vi "G#Interface_ExecuteVI.vi"(0 "reference in":refnum<class "G#Interface.lvclass">, 2 "VI Refnum":refnum<vi>, 5 "error in (no error)":errorcluster) -> (14 "reference out":refnum<class "G#Interface.lvclass">, 19 "error out":errorcluster)   [LabVIEW 2020, in "G#Interface.lvclass"]
uses:
  G#Interface.lvclass
  C:/ProjectGSharpDevelopment_2020-3/gsharp/VIPM/Files/vi.lib/addons/_AddQ/G#Object/G#Object.lvclass
  G#Interface.lvclass/G#Interface.ctl
  G#Object/G#Object.lvclass
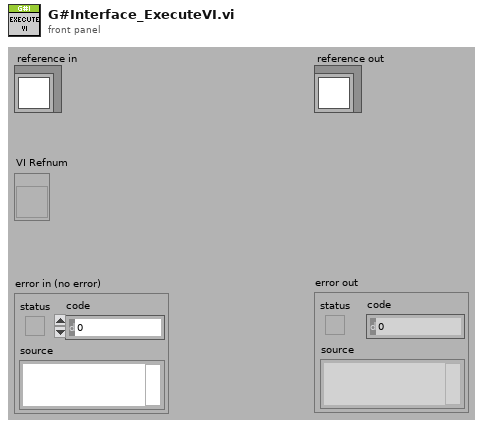
[diagram p1: front panel]
types:
  T1 = typedef "G#Object.lvclass/G#Object_ClassHierarchy.ctl" = cluster{"ClassName":string, "FullClassName":string, "ClassPath":path, "IsLeaf":bool}
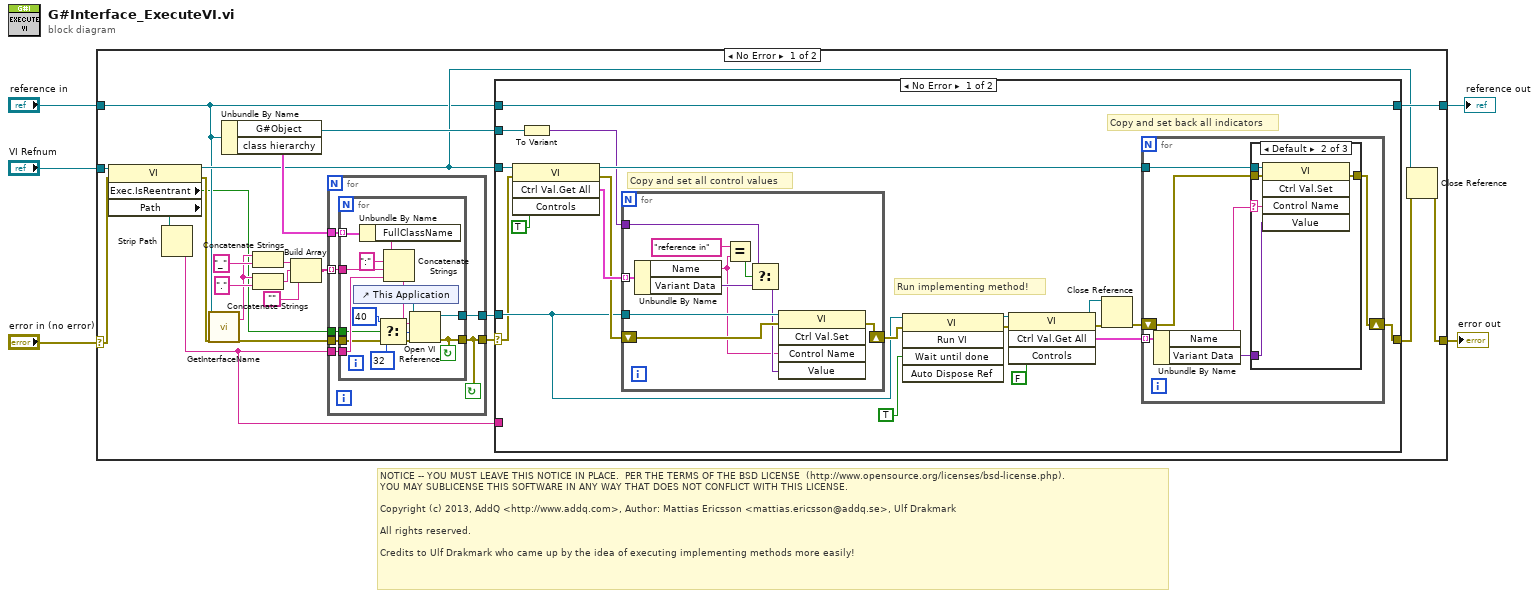
[diagram p0: block diagram]
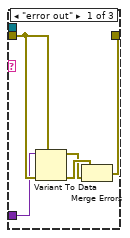
[diagram p2: hidden frame]
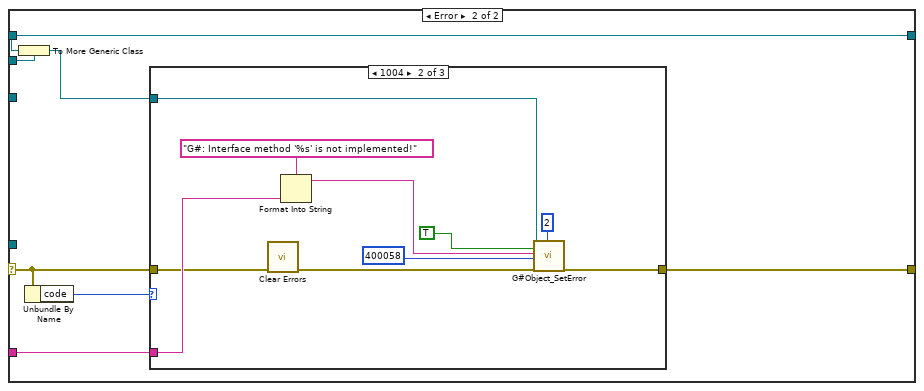
[diagram p4: hidden frame]
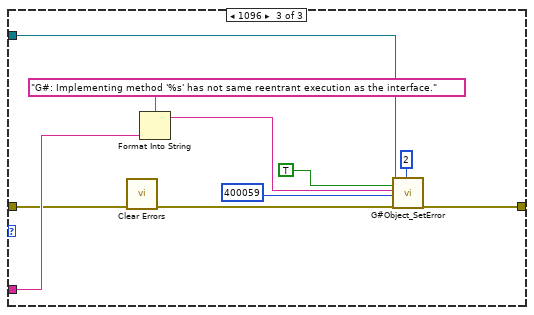
[diagram p6: hidden frame]
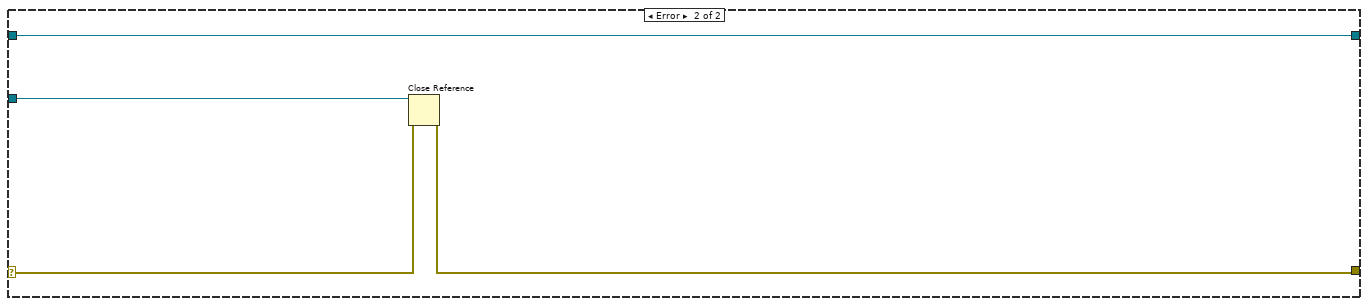
[diagram p7: hidden frame]
diagram:
  # "NOTICE -- YOU MUST LEAVE THIS NOTICE IN PLACE.  PER THE TERMS OF THE BSD LICENSE  (http://www.opensource.org/licenses/bsd-license.php).\nYOU MAY SUBLICENSE THIS SOFTWARE IN ANY WAY THAT DOES NOT CONFLICT WITH THIS LICENSE.\n\nCopyright (c) 2013, AddQ <http://www.addq.com>, Author: Mattias Ericsson <mattias.ericsson@addq.se>, Ulf Drakmark\n\nAll rights reserved.\n\nCredits to Ulf Drakmark who came up by the idea of executing implementing methods more easily!"
  n1 = case shown="No Error" "error in (no error)" {
    selector: "error in (no error)" -> [w27 w126]
    tunnel: "VI Refnum" -> [w28 w127]
    tunnel: "reference in" -> [w15 w128]
    tunnel: [w22 w128] -> w2
    tunnel: [w19 w125] -> w1
    frame No Error {
      n2 = property class="VI"(reference=w28, error in=w27) -> (reference out=w20:refnum<vi>, error out=w17:errorcluster, "Exec.IsReentrant"=w6:bool, "Path"=w7:path)
      n3 = Strip Path(path=w7) -> (name=w21:string)  [unwired: 1 out]
      n4 = call-dynamic "GetInterfaceName.vi"("reference in"=w15, "error in (no error)"=w17) -> ("interface name"=w12:string, "error out"=w16:errorcluster)  [unwired: 13 in, 3 out]
      n5 = Unbundle By Name(w15) -> ("G#Object"=w23:refnum<class "G#Object.lvclass">, "class hierarchy"=w26:T1[])
      n6 = Concatenate Strings(w12, "_" ("string")) -> (w11:string)
      n7 = Concatenate Strings(w12, "." ("string")) -> (w10:string)
      n8 = Build Array(w11, w10, "") -> (w8:string[])
      n9 = for {
        tunnel: w26 -> [w35]
        tunnel: [w34] -> w25
        tunnel: [w31] -> w24
        tunnel: w21 -> [w33]
        tunnel: w16 -> [w32]
        tunnel: w8 -> [w30] mode=indexing
        tunnel: w6 -> [w29]
        stop <- w31 continue-if-true
        n10 = for {
          tunnel: w35 -> [w49] mode=indexing
          tunnel: w33 -> [w47]
          tunnel: w32 -> [w45]
          tunnel: [w42] -> w31
          tunnel: [w41] -> w34
          tunnel: w30 -> [w40]
          tunnel: w29 -> [w36]
          stop <- w42 continue-if-true
          n11 = control-ref of="This Application"() -> (w43:refnum<vi>)
          n12 = Unbundle By Name(w49) -> ("FullClassName"=w48:string)
          n13 = Select(t=40 ("options"), s=w36, f=32 ("options")) -> (s? t:f=w38:i32)
          n14 = Concatenate Strings(w48, ":" ("string"), w40, w47) -> (w44:string)
          n15 = Open VI Reference(application reference (local)=w43, vi path=w44, options=w38, error in (no error)=w45) -> (vi reference=w41:refnum<vi>, error out=w42:errorcluster)  [unwired: 2 in]
        }
      }
      n16 = case shown="No Error" w24 {
        selector: w24 -> [w54 w98]
        tunnel: w20 -> [w69 _]
        tunnel: w23 -> [w52 w100]
        tunnel: w25 -> [w64 _]
        tunnel: [w50 w103] -> w18
        tunnel: w15 -> [w51 w101]
        tunnel: [w51 w101] -> w22
        tunnel: w21 -> [_ w102]
        frame No Error {
          # "Copy and set back all indicators"
          # "Run implementing method!"
          # "Copy and set all control values"
          n17 = invoke class="VI" method="Ctrl Val.Get All"(reference=w69, error in=w54, "Controls"=TRUE) -> (reference out=w58:refnum<vi>, error out=w66:errorcluster, "Get All Control Values Variant"=w67:cluster{"Name":string, "Variant Data":variant}[])  [unwired: 1 in, 1 out]
          n18 = To Variant(anything=w52) -> (Variant=w53:variant)
          n19 = for {
            tunnel: w67 -> [w96] mode=indexing
            tunnel: w53 -> [w95]
            tunnel: w64 -> [w91]
            shift-right: [w89] -> w65
            shift-left: w66 -> [w90]
            n20 = Unbundle By Name(w96) -> ("Name"=w87:string, "Variant Data"=w92:variant)
            n21 = Equal?(x="reference in" ("Name"), y=w87) -> (x = y?=w93:bool)
            n22 = Select(t=w95, s=w93, f=w92) -> (s? t:f=w88:variant)
            n23 = invoke class="VI" method="Ctrl Val.Set"(reference=w91, error in=w90, "Control Name"=w87, "Value"=w88) -> (error out=w89:errorcluster)  [unwired: 1 in, 4 out]
          }
          n24 = invoke class="VI" method="Run VI"(reference=w64, error in=w65, "Wait until done"=TRUE ("Wait Until Done")) -> (reference out=w61:refnum<vi>, error out=w62:errorcluster)  [unwired: 2 in, 3 out]
          n25 = invoke class="VI" method="Ctrl Val.Get All"(reference=w61, error in=w62, "Controls"=FALSE) -> (reference out=w56:refnum<vi>, error out=w57:errorcluster, "Get All Control Values Variant"=w59:cluster{"Name":string, "Variant Data":variant}[])  [unwired: 1 in, 1 out]
          n26 = Close Reference(reference=w56, error in (no error)=w57) -> (error out=w55:errorcluster)
          n27 = for {
            tunnel: w58 -> [w75]
            tunnel: w59 -> [w73] mode=indexing
            shift-right: [w70] -> w50
            shift-left: w55 -> [w74]
            n28 = Unbundle By Name(w73) -> ("Name"=w72:string, "Variant Data"=w71:variant)
            n29 = case shown="Default" w72 {
              selector: w72 -> [_ w83 _]
              tunnel: w75 -> [_ w85 _]
              tunnel: w74 -> [w80 w84 w86]
              tunnel: w71 -> [w79 w82 _]
              tunnel: [w76 w81 w86] -> w70
              frame "error out" {
                n30 = Variant To Data(error in=w80, type=w80, Variant=w79) -> (data=w77:errorcluster, error out=w78:errorcluster)
                n31 = Merge Errors(w78, w77) -> (w76:errorcluster)
              }
              frame Default {
                n32 = invoke class="VI" method="Ctrl Val.Set"(reference=w85, error in=w84, "Control Name"=w83, "Value"=w82) -> (error out=w81:errorcluster)  [unwired: 1 in, 4 out]
              }
              frame "reference out" {
                # "Do not update\nreference out"
              }
            }
          }
        }
        frame Error {
          n33 = To More Generic Class(target class=w100, reference=w101) -> (generic class reference=w99:refnum<class "G#Object.lvclass">)
          n34 = Unbundle By Name(w98) -> ("code"=w97:i32)
          n35 = case shown="1004" w97 {
            tunnel: [w104 w112 w122] -> w103
            tunnel: w102 -> [_ w109 w119]
            tunnel: w99 -> [_ w106 w116]
            tunnel: w98 -> [w104 w105 w115]
            frame Default {
            }
            frame 1004 {
              n36 = call <vilib>:"Clear Errors.vi"("error in (no error)"=w105) -> ("error out"=w114:errorcluster)  [unwired: 5 in, 1 out]
              n37 = Format Into String(format string="G#: Interface method '%s' is not implemented!", w109) -> (resulting string=w107:string)  [unwired: 2 in, 1 out]
              n38 = call "G#Object_SetError.vi"("reference in"=w106, "error (F)"=TRUE, "source"=w107, "code"=400058, "error in (no error)"=w114, "call depth (1)"=2) -> ("error out"=w112:errorcluster)  [unwired: 13 in]
            }
            frame 1096 {
              n39 = call <vilib>:"Clear Errors.vi"("error in (no error)"=w115) -> ("error out"=w124:errorcluster)  [unwired: 5 in, 1 out]
              n40 = Format Into String(format string="G#: Implementing method '%s' has not same reentrant execution as the interface.", w119) -> (resulting string=w117:string)  [unwired: 2 in, 1 out]
              n41 = call "G#Object_SetError.vi"("reference in"=w116, "error (F)"=TRUE, "source"=w117, "code"=400059, "error in (no error)"=w124, "call depth (1)"=2) -> ("error out"=w122:errorcluster)  [unwired: 13 in]
            }
          }
        }
      }
      n42 = Close Reference(reference=w20, error in (no error)=w18) -> (error out=w19:errorcluster)
    }
    frame Error {
      n43 = Close Reference(reference=w127, error in (no error)=w126) -> (error out=w125:errorcluster)
    }
  }
  "error out" <- w1
  "reference out" <- w2
